vi "VNS IRH3T.vi"() -> ()   [LabVIEW 2013]
uses:
  Classes/OSSP_Problem.lvclass
  Classes/OSSP_Problem.lvclass/OSSP_Problem.ctl
  Classes/Scheduler_Class/Prins FIFO Scheduler Methods and Controls/Prins FIFO Scheduler.vi
  Classes/Scheduler_Class/Prins FIFO Scheduler Methods and Controls/Methods/Calculate Final Completion Times of Jobs.vi
  Classes/Scheduler_Class/Prins FIFO Scheduler Methods and Controls/Methods/Reorder Schedule(Prins FIFO) based on Start Times.vi
  GA/SubVIS/Remove Duplicates In Array.vi
  GA/SubVIS/Calcualte General Tardiness.vi
  Classes/Scheduler_Class/Prins FIFO Scheduler Methods and Controls/Methods/UpdateMachineGaps.vi
  Classes/Scheduler_Class/Prins FIFO Scheduler Methods and Controls/Methods/UpdateJobGaps.vi
  Classes/Scheduler_Class/Prins FIFO Scheduler Methods and Controls/Methods/Find Intersecting Gaps.vi
  <vilib>/Analysis/1siggen.llb/Riffle Array (I32).vi
  Classes/Scheduler_Class/Prins FIFO Scheduler Methods and Controls/Methods/Transform to Plain Job and Machine Gaps Array.vi
  <vilib>/Analysis/NI_AALBase.lvlib
  Classes/Scheduler.lvclass
panel:
  in  "Problem Type":enum16{"Taillard", "Brucker", "Gueret Prins"}(ring)
  in  "Instance Number for Taillard":dbl
  out "Tardiness(FIFO Engine)":u16
  out "VNS Result":u16[](array[numeric])
  out "Best Chromosome":i32[](array[numeric])
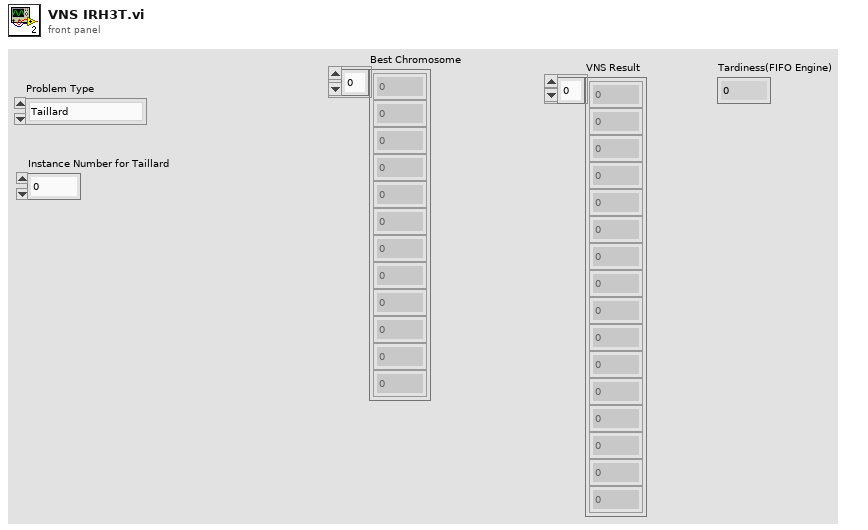
[diagram p1: front panel]
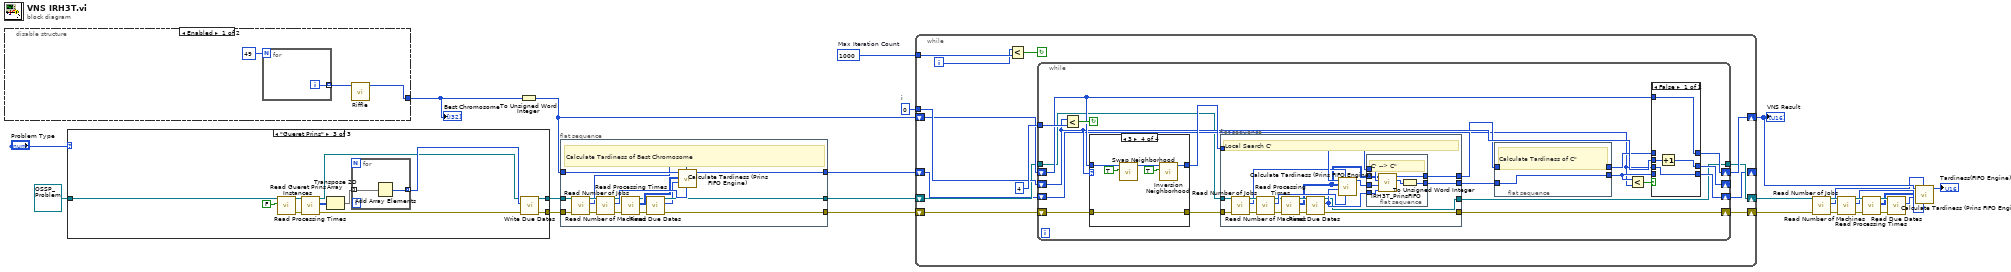
[diagram p0: block diagram]
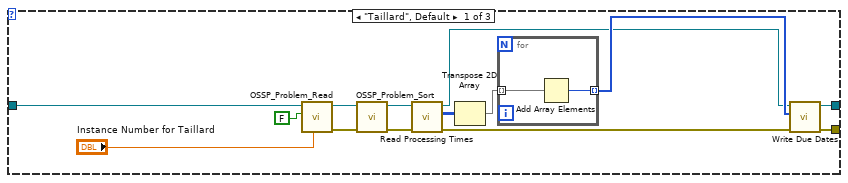
[diagram p2: hidden frame]
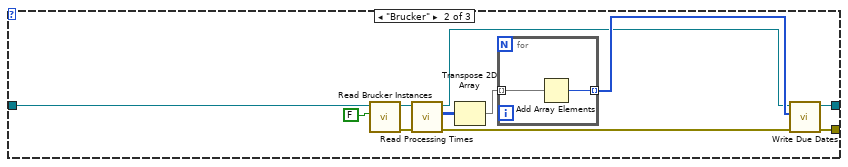
[diagram p3: hidden frame]
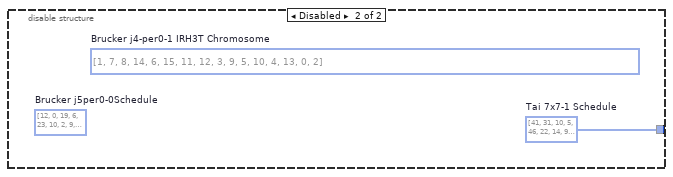
[diagram p4: hidden frame]
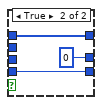
[diagram p5: hidden frame]
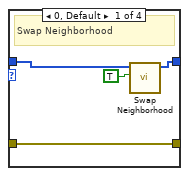
[diagram p6: hidden frame]
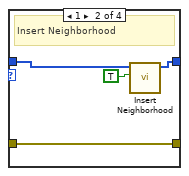
[diagram p7: hidden frame]
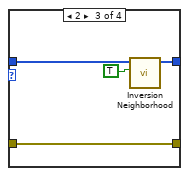
[diagram p8: hidden frame]
diagram:
  w24 = 0  # i
  w25 = 1000  # Max Iteration Count
  n1 = disable-structure shown="Enabled" {
    disable-tunnel: [w26 w30] -> w23
    frame Enabled {
      n2 = for {
        N: 49 -> [_]
        tunnel: [w29] -> w27 mode=indexing
        i -> [w29]
      }
      n3 = call-poly <vilib>:"Riffle.vi"("X"=w27) -> ("Riffled {X}"=w26:i32[])  [unwired: 8 in, 2 out]
    }
    frame Disabled {
      w30 = i32[] [41, 31, 10, 5, 46, 22, 14, 9, 30, 39, 48, 21, 15, 3, 12, 34, 44, 32, 35, 27, 0, 38, 17, 36, 19, 8, 45, 37, 11, 29, 1, 28, 18, 16, 40, 23, 24, 13, 4, 43, 33, 7, 6, 25, 47, 2, 20, 42, 26]  # Tai 7x7-1 Schedule
      (unwired) i32[] [12, 0, 19, 6, 23, 10, 2, 9, 16, 8, 24, 11, 15, 7, 3, 20, 14, 18, 1, 5, 22, 13, 17, 21, 4]  # Brucker j5per0-0Schedule
      (unwired) i32[] [1, 7, 8, 14, 6, 15, 11, 12, 3, 9, 5, 10, 4, 13, 0, 2]  # Brucker j4-per0-1 IRH3T Chromosome
    }
  }
  "Best Chromosome" <- w23
  n4 = case shown="\"Gueret Prins\"" "Problem Type" {
    tunnel: refnum<class "OSSP_Problem.lvclass"> refnum ("OSSP_Problem.lvclass") -> [w44 w57 w70]
    tunnel: [w37 w52 w65] -> w18
    tunnel: [w36 w53 w66] -> w6
    frame "Taillard", Default {
      n5 = call "OSSP_Problem_Read.vi"("Instance Number"="Instance Number for Taillard", "Auto Mode"=FALSE, "OSSP_Problem.lvclass In"=w44) -> ("error out"=w41:errorcluster, "OSSP_Problem.lvclass Out"=w42:refnum<class "OSSP_Problem.lvclass">)  [unwired: 7 in]
      n6 = call "OSSP_Problem_Sort.vi"("error in (no error)"=w41, "OSSP_Problem.lvclass In"=w42) -> ("error out"=w39:errorcluster, "OSSP_Problem.lvclass Out"=w38:refnum<class "OSSP_Problem.lvclass">)  [unwired: 8 in]
      n7 = call "Read Processing Times.vi"("error in (no error)"=w39, "OSSP_Problem in"=w38) -> ("error out"=w31:errorcluster, "Processing Times"=w34:u16[][], "OSSP_Problem out"=w32:refnum<class "OSSP_Problem.lvclass">)  [unwired: 7 in]
      n8 = Transpose 2D Array(2D array=w34) -> (transposed array=w35:u16[][])
      n9 = for {
        tunnel: w35 -> [w46] mode=indexing
        tunnel: [w45] -> w33 mode=indexing
        n10 = Add Array Elements(numeric array=w46) -> (sum=w45:u16)
      }
      n11 = call "Write Due Dates.vi"("error in (no error)"=w31, "Due Dates"=w33, "OSSP_Problem in"=w32) -> ("error out"=w36:errorcluster, "OSSP_Problem out"=w37:refnum<class "OSSP_Problem.lvclass">)  [unwired: 7 in]
    }
    frame "Brucker" {
      n12 = call "Read Brucker Instances.vi"("Auto Mode"=FALSE, "OSSP_Problem in"=w57) -> ("error out"=w54:errorcluster, "OSSP_Problem out"=w55:refnum<class "OSSP_Problem.lvclass">)  [unwired: 8 in]
      n13 = call "Read Processing Times.vi"("error in (no error)"=w54, "OSSP_Problem in"=w55) -> ("error out"=w47:errorcluster, "Processing Times"=w50:u16[][], "OSSP_Problem out"=w48:refnum<class "OSSP_Problem.lvclass">)  [unwired: 7 in]
      n14 = Transpose 2D Array(2D array=w50) -> (transposed array=w51:u16[][])
      n15 = for {
        tunnel: w51 -> [w59] mode=indexing
        tunnel: [w58] -> w49 mode=indexing
        n16 = Add Array Elements(numeric array=w59) -> (sum=w58:u16)
      }
      n17 = call "Write Due Dates.vi"("error in (no error)"=w47, "Due Dates"=w49, "OSSP_Problem in"=w48) -> ("error out"=w53:errorcluster, "OSSP_Problem out"=w52:refnum<class "OSSP_Problem.lvclass">)  [unwired: 7 in]
    }
    frame "Gueret Prins" {
      n18 = call "Read Gueret Prins Instances.vi"("Auto Mode"=FALSE, "OSSP_Problem in"=w70) -> ("error out"=w67:errorcluster, "OSSP_Problem out"=w68:refnum<class "OSSP_Problem.lvclass">)  [unwired: 8 in]
      n19 = call "Read Processing Times.vi"("error in (no error)"=w67, "OSSP_Problem in"=w68) -> ("error out"=w60:errorcluster, "Processing Times"=w63:u16[][], "OSSP_Problem out"=w61:refnum<class "OSSP_Problem.lvclass">)  [unwired: 7 in]
      n20 = Transpose 2D Array(2D array=w63) -> (transposed array=w64:u16[][])
      n21 = for {
        tunnel: w64 -> [w72] mode=indexing
        tunnel: [w71] -> w62 mode=indexing
        n22 = Add Array Elements(numeric array=w72) -> (sum=w71:u16)
      }
      n23 = call "Write Due Dates.vi"("error in (no error)"=w60, "Due Dates"=w62, "OSSP_Problem in"=w61) -> ("error out"=w66:errorcluster, "OSSP_Problem out"=w65:refnum<class "OSSP_Problem.lvclass">)  [unwired: 7 in]
    }
  }
  n24 = To Unsigned Word Integer(number=w23) -> (unsigned 16bit integer=w17:u16[])
  n25 = flat-sequence {
    tunnel: w17 -> [w88]
    tunnel: [w87] -> w16
    tunnel: w18 -> [w86]
    tunnel: [w79] -> w15
    tunnel: w6 -> [w77]
    tunnel: [w73] -> w5
    frame #0 {
      # "Calculate Tardiness of Best Chromosome"
      n26 = call "Read Number of Jobs.vi"("error in (no error)"=w77, "OSSP_Problem in"=w86) -> ("error out"=w76:errorcluster, "Number of Jobs"=w84:i32, "OSSP_Problem out"=w85:refnum<class "OSSP_Problem.lvclass">)  [unwired: 7 in]
      n27 = call "Read Number of Machines.vi"("error in (no error)"=w76, "OSSP_Problem in"=w85) -> ("error out"=w75:errorcluster, "Number of Machines"=w83:i32, "OSSP_Problem out"=w82:refnum<class "OSSP_Problem.lvclass">)  [unwired: 7 in]
      n28 = call "Read Processing Times.vi"("error in (no error)"=w75, "OSSP_Problem in"=w82) -> ("error out"=w74:errorcluster, "Processing Times"=w81:u16[][], "OSSP_Problem out"=w80:refnum<class "OSSP_Problem.lvclass">)  [unwired: 7 in]
      n29 = call "Read Due Dates.vi"("error in (no error)"=w74, "OSSP_Problem in"=w80) -> ("error out"=w73:errorcluster, "Due Dates"=w78:u16[], "OSSP_Problem out"=w79:refnum<class "OSSP_Problem.lvclass">)  [unwired: 7 in]
      n30 = call "Calculate Tardiness (Prins FIFO Engine).vi"("Number of Machines"=w83, "Number of Jobs"=w84, "Due Dates"=w78, "Processing Times"=w81, "Schedule In"=w88) -> ("Tardiness(Prins FIFO Engine)"=w87:u16)  [unwired: 5 in, 1 out]
    }
  }
  n31 = while {
    tunnel: w25 -> [w101]
    tunnel: w24 -> [w98]
    shift-right: [w96] -> w22
    shift-left: w17 -> [w95]
    shift-right: [w94] -> w14
    shift-left: w15 -> [w93]
    shift-right: [w92] -> _
    shift-left: w16 -> [w91]
    shift-right: [w89] -> w4
    shift-left: w5 -> [w90]
    i -> [w97]
    stop <- w100 continue-if-true
    n32 = Less?(x=w97, y=w101) -> (x < y?=w100:bool)
    n33 = while {
      tunnel: 4 -> [w117]
      shift-right: [w116] -> _
      shift-left: w98 -> [w113]
      shift-right: [w115] -> w96
      shift-left: w95 -> [w114]
      shift-right: [w108] -> w92
      shift-left: w91 -> [w107]
      tunnel: w93 -> [w106]
      tunnel: [w105] -> w94
      shift-right: [w102] -> w89
      shift-left: w90 -> [w104]
      stop <- w120 continue-if-true
      n34 = Less?(x=w113, y=w117) -> (x < y?=w120:bool)
      n35 = case shown="3" w113 {
        tunnel: w114 -> [w158 w162 w166 w172]
        tunnel: [w157 w161 w165 w170] -> w119
        tunnel: w104 -> [w155 w159 w163 w167]
        tunnel: [w155 w159 w163 w167] -> w103
        frame 0, Default {
          # "Swap Neighborhood"
          n36 = call "Swap Neighborhood.vi"("Generate Random Indices?"=TRUE, "Schedule In"=w158) -> ("Schedule Out"=w157:u16[])  [unwired: 9 in]
        }
        frame 1 {
          # "Insert Neighborhood"
          n37 = call "Insert Neighborhood.vi"("Generate Random Indices?"=TRUE, "C'"=w162) -> ("Chromosome Out"=w161:u16[])  [unwired: 9 in]
        }
        frame 2 {
          n38 = call "Inversion Neighborhood.vi"("Generate Random Indices?"=TRUE, "Schedule in"=w166) -> ("Schedule out"=w165:u16[])  [unwired: 9 in]
        }
        frame 3 {
          n39 = call "Swap Neighborhood.vi"("Generate Random Indices?"=TRUE, "Schedule In"=w172) -> ("Schedule Out"=w171:u16[])  [unwired: 9 in]
          n40 = call "Inversion Neighborhood.vi"("Generate Random Indices?"=TRUE, "Schedule in"=w171) -> ("Schedule out"=w170:u16[])  [unwired: 9 in]
        }
      }
      n41 = flat-sequence {
        tunnel: w119 -> [w146]
        tunnel: [w147] -> w111
        tunnel: [w144] -> w112
        tunnel: w106 -> [w143]
        tunnel: [w135] -> w105
        tunnel: w103 -> [w134]
        tunnel: [w130] -> w102
        frame #0 {
          # "Local Search C'"
          n42 = call "Read Number of Jobs.vi"("error in (no error)"=w134, "OSSP_Problem in"=w143) -> ("error out"=w133:errorcluster, "Number of Jobs"=w141:i32, "OSSP_Problem out"=w142:refnum<class "OSSP_Problem.lvclass">)  [unwired: 7 in]
          n43 = call "Read Number of Machines.vi"("error in (no error)"=w133, "OSSP_Problem in"=w142) -> ("error out"=w132:errorcluster, "Number of Machines"=w140:i32, "OSSP_Problem out"=w139:refnum<class "OSSP_Problem.lvclass">)  [unwired: 7 in]
          n44 = call "Read Processing Times.vi"("error in (no error)"=w132, "OSSP_Problem in"=w139) -> ("error out"=w131:errorcluster, "Processing Times"=w136:u16[][], "OSSP_Problem out"=w138:refnum<class "OSSP_Problem.lvclass">)  [unwired: 7 in]
          n45 = call "Read Due Dates.vi"("error in (no error)"=w131, "OSSP_Problem in"=w138) -> ("error out"=w130:errorcluster, "Due Dates"=w137:u16[], "OSSP_Problem out"=w135:refnum<class "OSSP_Problem.lvclass">)  [unwired: 7 in]
          n46 = call "Calculate Tardiness (Prins FIFO Engine).vi"("Number of Machines"=w140, "Number of Jobs"=w141, "Due Dates"=w137, "Processing Times"=w136, "Schedule In"=w146) -> ("Tardiness(Prins FIFO Engine)"=w145:u16)  [unwired: 5 in, 1 out]
          n47 = flat-sequence {
            tunnel: w146 -> [w154]
            tunnel: [w148] -> w147
            tunnel: w145 -> [w153]
            tunnel: w136 -> [w152]
            tunnel: w137 -> [w151]
            tunnel: [w149] -> w144
            frame #0 {
              # "C' --> C\""
              n48 = call "IRH3T_PrinsFIFO.vi"("Due Dates"=w151, "Initial Tardiness"=w153, "Schedule 2B Improved"=w154, "Proocessing Times  (Machines x Jobs)"=w152) -> ("Total Tardiness"=w150:u16, "IRH3T (Reordered) Schedule Out"=w148:u16[])  [unwired: 5 in, 1 out]
              n49 = To Unsigned Word Integer(number=w150) -> (unsigned 16bit integer=w149:u16)
            }
          }
        }
      }
      n50 = flat-sequence {
        tunnel: w111 -> [w121]
        tunnel: [w122] -> w109
        tunnel: w112 -> [w122]
        tunnel: [w121] -> w110
        frame #0 {
          # "Calculate Tardiness of C\""
        }
      }
      n51 = Less?(x=w109, y=w107) -> (x < y?=w118:bool)
      n52 = case shown="False" w118 {
        tunnel: w113 -> [w125 _]
        tunnel: w110 -> [_ w128]
        tunnel: [w126 0] -> w116
        tunnel: [w124 w128] -> w115
        tunnel: w114 -> [w124 _]
        tunnel: w109 -> [_ w127]
        tunnel: [w123 w127] -> w108
        tunnel: w107 -> [w123 _]
        frame False {
          n53 = Increment(x=w125) -> (x+1=w126:i32)
        }
        frame True {
        }
      }
    }
  }
  "VNS Result" <- w22
  n54 = call "Read Number of Jobs.vi"("error in (no error)"=w4, "OSSP_Problem in"=w14) -> ("error out"=w3:errorcluster, "Number of Jobs"=w10:i32, "OSSP_Problem out"=w13:refnum<class "OSSP_Problem.lvclass">)  [unwired: 7 in]
  n55 = call "Read Number of Machines.vi"("error in (no error)"=w3, "OSSP_Problem in"=w13) -> ("error out"=w2:errorcluster, "Number of Machines"=w9:i32, "OSSP_Problem out"=w12:refnum<class "OSSP_Problem.lvclass">)  [unwired: 7 in]
  n56 = call "Read Processing Times.vi"("error in (no error)"=w2, "OSSP_Problem in"=w12) -> ("error out"=w1:errorcluster, "Processing Times"=w8:u16[][], "OSSP_Problem out"=w11:refnum<class "OSSP_Problem.lvclass">)  [unwired: 7 in]
  n57 = call "Read Due Dates.vi"("error in (no error)"=w1, "OSSP_Problem in"=w11) -> ("Due Dates"=w7:u16[])  [unwired: 7 in, 2 out]
  n58 = call "Calculate Tardiness (Prins FIFO Engine).vi"("Number of Machines"=w9, "Number of Jobs"=w10, "Due Dates"=w7, "Processing Times"=w8, "Schedule In"=w22) -> ("Tardiness(Prins FIFO Engine)"=→"Tardiness(FIFO Engine)":u16)  [unwired: 5 in, 1 out]
